vi "TSP-Link Get Global.vi"(6 "Remote Variable Name":string, 7 "Local Variable Name":string, 8 "error in":errorcluster, 10 "Node In":string, 11 "VISA resource name":refnum<visa-resource-name>) -> (0 "error out":errorcluster, 2 "Node Out":string, 3 "VISA resource name out":refnum<visa-resource-name>, 4 "Command String":string)   [LabVIEW 2013, in "Keithley 2600 Series.lvlib"]
doc: "This VI gets the value of a variable on a remote node and copies it to a variable on the local node.\n\n<b>Remarks:</b>\nThis VI does not return the value of the variable on the remote node. Use one of the print commands on the local variable that was assigned the remote value to return the value.\n\n<b>Functions and Attributes Used</b>\nlocalnode.getglobal()\n\nNote: localnode is an artifact of command organization and is not a valid node name for use with this command.\n\nTSP-Link feature is not supported with Keithley 2604B, 2614B, 2634B."
uses:
  Keithley 2600 Series.lvlib
  Private/GlobalVariables.vi
panel:
  # "(c) 2008 Keithley Instruments, Inc.  ALL RIGHTS RESERVED."
  # ")"
  # "= node[x].getglobal("
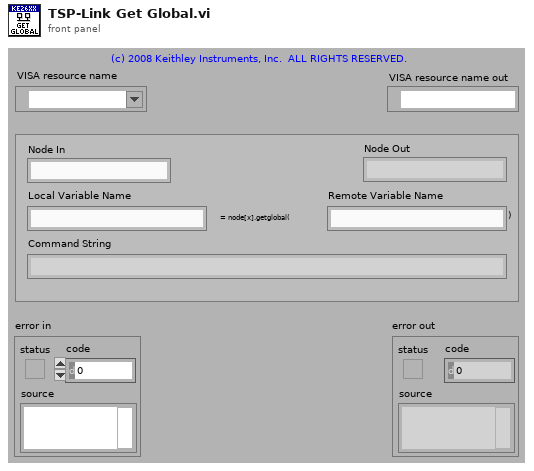
[diagram p1: front panel]
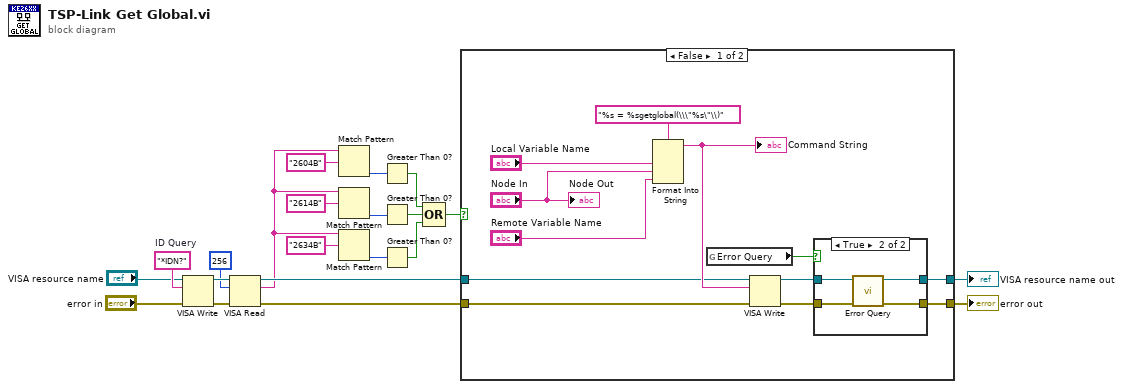
[diagram p0: block diagram]
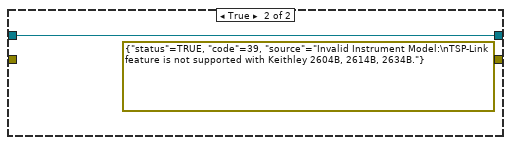
[diagram p3: hidden frame]
diagram:
  w16 = "*IDN?"  # ID Query
  n1 = VISA Write(VISA resource name="VISA resource name", write buffer=w16, error in (no error)="error in") -> (VISA resource name out=w19:refnum<visa-resource-name>, error out=w18:errorcluster)  [unwired: 1 out]
  n2 = VISA Read(VISA resource name=w19, byte count=u32 256, error in (no error)=w18) -> (VISA resource name out=w13:refnum<visa-resource-name>, read buffer=w2:string, error out=w12:errorcluster)  [unwired: 1 out]
  n3 = Match Pattern(string=w2, regular expression="2604B" ("y")) -> (offset past match=w8:i32)  [unwired: 1 in, 3 out]
  n4 = Match Pattern(string=w2, regular expression="2614B" ("y")) -> (offset past match=w7:i32)  [unwired: 1 in, 3 out]
  n5 = Match Pattern(string=w2, regular expression="2634B" ("y")) -> (offset past match=w6:i32)  [unwired: 1 in, 3 out]
  n6 = Greater Than 0?(x=w8) -> (x > 0?=w5:bool)
  n7 = Greater Than 0?(x=w7) -> (x > 0?=w4:bool)
  n8 = Greater Than 0?(x=w6) -> (x > 0?=w3:bool)
  n9 = Compound Arithmetic op=OR(w5, w4, w3) -> (w1:bool)
  n10 = case shown="False" w1 {
    tunnel: [w26 w41] -> w21
    tunnel: [w25 errorcluster {"status"=TRUE, "code"=39, "source"="Invalid Instrument Model:\nTSP-Link feature is not supported with Keithley 2604B, 2614B, 2634B."} ("error out")] -> w20
    tunnel: w13 -> [w23 w41]
    tunnel: w12 -> [w22 _]
    frame False {
      n11 = Format Into String(format string="%s = %sgetglobal(\\\"%s\"\\)", "Local Variable Name", "Node In", "Remote Variable Name") -> (resulting string=w24:string)  [unwired: 2 in, 1 out]
      "Command String" <- w24
      n12 = global read "GlobalVariables.vi" "Error Query"() -> (w29:bool)
      n13 = VISA Write(VISA resource name=w23, write buffer=w24, error in (no error)=w22) -> (VISA resource name out=w28:refnum<visa-resource-name>, error out=w27:errorcluster)  [unwired: 1 out]
      n14 = case shown="True" w29 {
        tunnel: w28 -> [w35 w39]
        tunnel: w27 -> [w34 w38]
        tunnel: [w35 w37] -> w26
        tunnel: [w34 w36] -> w25
        frame False {
        }
        frame True {
          n15 = call "Error Query.vi"("error in (no error)"=w38, "VISA resource name"=w39) -> ("error out"=w36:errorcluster, "VISA resource name out"=w37:refnum<visa-resource-name>)  [unwired: 8 out]
        }
      }
      "Node Out" <- "Node In"
    }
    frame True {
    }
  }
  "VISA resource name out" <- w21
  "error out" <- w20
